vi "Pre Launch Init.vi"(11 "Digital Input in":refnum<class "Digital Input.lvclass">) -> (0 "error out":errorcluster, 3 "Digital Input out":refnum<class "Digital Input.lvclass">)   [LabVIEW 2021, in "Digital Input.lvlib" / "Digital Input.lvclass"]
doc: "(<B>Filename</B>: Actor Framework.lvlib:Actor.lvclass:Pre Launch Init.vi)\n\nDefines behavior that occurs after the Launch Nested Actor method is invoked but before the actor's Actor Core method begins running.\n\nBy default, this method does nothing. A descendant class may override it to define behavior."
uses:
  Digital Input.lvclass
  Digital Input.lvclass/Digital Input.ctl
  <vilib>/ActorFramework/Message Enqueuer/Init from Existing Queue.vi
  <vilib>/DAQmx/configure/timing.llb/DAQmx Timing (Sample Clock).vi
  <vilib>/ActorFramework/Actor/Actor.lvclass
  <vilib>/ActorFramework/Message Enqueuer/Message Enqueuer.lvclass
  Digital Input Messages/Acquire Digital Msg/Acquire Digital Msg.lvclass
  C:/Program Files/National Instruments/LabVIEW 2021/vi.lib/ActorFramework/Actor/Actor.lvclass
  C:/git/Digital-Tasks/Digital Input/Digital Input/Digital Input/Digital Input.lvclass
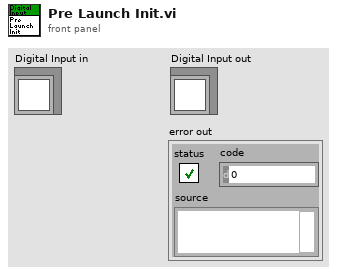
[diagram p1: front panel]
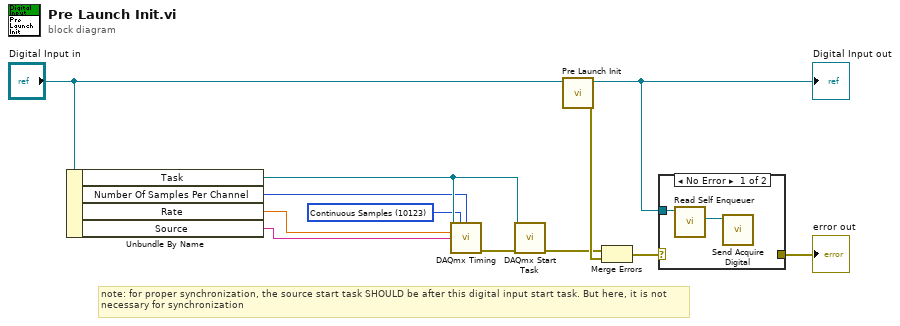
[diagram p0: block diagram]
diagram:
  w6 = 10123 items=["Finite Samples"=10178, "Continuous Samples"=10123, "Hardware Timed Single Point"=12522] ("sample mode")
  # "note: for proper synchronization, the source start task SHOULD be after this digital input start task. But here, it is not necessary for synchronization"
  n1 = Unbundle By Name("Digital Input in") -> ("Task"=w9:refnum<k21>, "Number Of Samples Per Channel"=w5:i32, "Rate"=w11:dbl, "Source"=w10:tag)
  n2 = call-poly <vilib>:"DAQmx Timing.vi"("task/channels in"=w9, "sample mode"=w6, "samples per channel"=w5, "rate"=w11, "source"=w10) -> ("error out"=w7:errorcluster)  [unwired: 9 in, 1 out]
  n3 = call <vilib>:"DAQmx Start Task.vi"("task/channels in"=w9, "error in"=w7) -> ("error out"=w4:errorcluster)  [unwired: 12 in, 1 out]
  n4 = call-parent "Pre Launch Init.vi"("Actor in"="Digital Input in") -> ("error out"=w12:errorcluster, "Actor out"=w1:refnum<class "Digital Input.lvclass">)  [unwired: 9 in]
  "Digital Input out" <- w1
  n5 = Merge Errors(w4, w12) -> (w3:errorcluster)
  n6 = case shown="No Error" w3 {
    selector: w3 -> [_ w15]
    tunnel: [_ w15] -> w2
    tunnel: w1 -> [w14 _]
    frame No Error {
      n7 = call <vilib>:"Read Self Enqueuer.vi"("Actor"=w14) -> ("Self Enqueuer"=w13:refnum<class "Message Enqueuer.lvclass">)  [unwired: 10 in]
      n8 = call "Send Acquire Digital.vi"("Message Enqueuer"=w13) -> ()  [unwired: 9 in, 2 out]
    }
    frame Error {
    }
  }
  "error out" <- w2
